vi "Analog Output.vi"() -> ()   [LabVIEW 2025]
doc: "Analog Output Example\n\nThis example will write the Output Voltage value to one of two analog output channels on the MXP port of the roboRIO.\n\nThis example expects a USB cable connected from your development PC to the Type B USB Jack (next to the power input) on the roboRIO."
uses:
  <vilib>/Rock Robotics/WPI/AnalogOutput/WPI_AnalogOutputChannel.ctl
panel:
  in  "AO Channel":T1
  in  "Output Voltage":dbl(slide) scale=0.0..6.0
  in  "stop":bool
  # "Set this input before running."
  # "This can be set while running."
  # "roboRIO Wiring"
  # "Analog Out 0"
  # "AO 0 = MXP pin 2\nAO 1 = MXP pin 4\nGND = MXP pins 6,8,12,16,20,24,28,30"
  # "Ground"
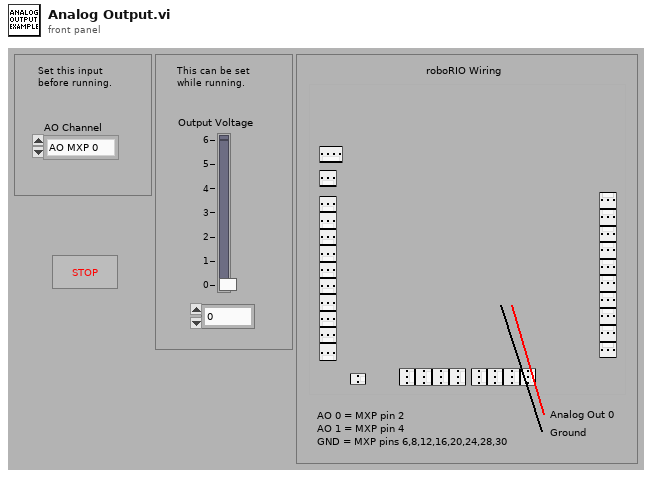
[diagram p1: front panel]
types:
  T1 = typedef "WPI_AnalogOutputChannel.ctl" = enum8{"AO MXP 0", "AO MXP 1", "Invalid"}
  T2 = typedef "WPI_AOChannelDevRef.ctl" = cluster{"DevStatus":errorcluster, "AO Channel":T1}
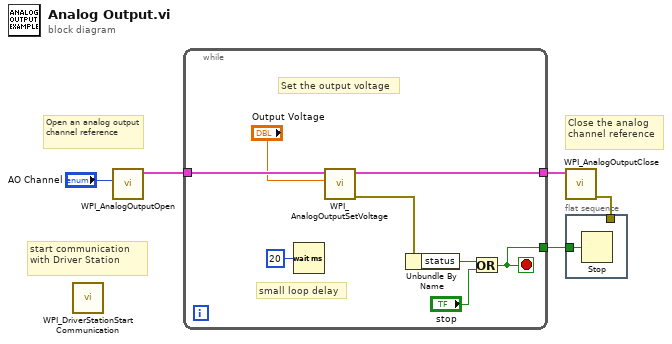
[diagram p0: block diagram]
diagram:
  # "start communication with Driver Station"
  # "Close the analog\nchannel reference"
  # "Open an analog output channel reference"
  n1 = call <vilib>:"WPI_DriverStationStart Communication.vi"() -> ()  [unwired: 3 in, 9 out]
  n2 = call <vilib>:"WPI_AnalogOutputOpen.vi"("AO Channel"="AO Channel") -> ("AODeviceRef"=w5:T2)  [unwired: 9 in, 1 out]
  n3 = while {
    tunnel: w5 -> [w9]
    tunnel: [w7] -> w4
    tunnel: [w10] -> w3
    stop <- w10 stop-if-true
    # "small loop delay"
    # "Set the output voltage"
    n4 = Wait (ms)(milliseconds to wait=u32 20) -> ()  [unwired: 1 out]
    n5 = call <vilib>:"WPI_AnalogOutputSetVoltage.vi"("Voltage"="Output Voltage", "AODeviceRef"=w9) -> ("error out"=w8:errorcluster, "AODeviceRef"=w7:T2)  [unwired: 8 in]
    n6 = Unbundle By Name(w8) -> ("status"=w12:bool)
    n7 = Or(x=w12, y="stop") -> (x .or. y?=w10:bool)
  }
  n8 = call <vilib>:"WPI_AnalogOutputClose.vi"("AODeviceRef"=w4) -> ("error out"=w2:errorcluster)  [unwired: 10 in]
  n9 = flat-sequence {
    tunnel: w3 -> [w14]
    tunnel: w2 -> [_]
    frame #0 {
      n10 = Stop(stop? (T)=w14) -> ()
    }
  }
